vi "read (lakeshore).vi"(0 "error in (no error)":errorcluster) -> (1 "read buffer":string, 2 "error out":errorcluster)   [LabVIEW 2011]
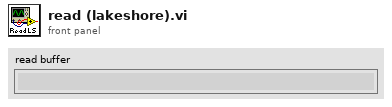
[diagram p1: front panel]
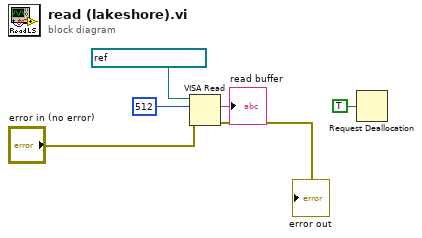
[diagram p0: block diagram]
diagram:
  n1 = VISA Read(VISA resource name=refnum<visa-resource-name> "GPIB0::12::INSTR", byte count=u32 512, error in (no error)="error in (no error)") -> (read buffer=→"read buffer":string, error out=→"error out":errorcluster)  [unwired: 2 out]
  n2 = Request Deallocation(TRUE ("flag")) -> ()
